vi "5ChTrigs_ABUT.vi"(4 "xmit ring":i32 min=0 max=4 step=1, 5 "Trans Geometry (mm)":T1={"Transducer"=0, "Geo Focus"=12.0, "a (radius)"=3.0, "# of rings"=5, "kerf space "=0.1, "Center Freq"=12.0} {"Transducer" items=["6D 12R 40 MHz"=0, "10D 31R 20 MHz"=1, "10D 23R 20 MHz"=2, "6D 23R 40 MHz"=3, "4.5D 10.7R 40 MHz"=4, "9D 23.5R 20 MHz"=5, "9D 25.8R 20MHz"=6, "Enter"=99]}, 6 "Digitizer Settings":T3={"Digitizer delay (us) "=0.0, "rf points per line"=2048, "lines per plane"=128, "Samp Rate (Hz)"=100000000.0, "Additional dig delay (us)"=0.0, "Voltage Scale"=0.4, "Pre-Looks"=0, "Offset delay (us)"=0.0, "bits A/D"=8, "Avg Num"=1, "DigTimeOut"=5.0, "Rel Dig Delay"=0.0, "Dig Ch"=0, "LeCroyCluster"={"LeCroy Channels"=[TRUE, FALSE, FALSE, FALSE], "LC read pt offset"=0.0, "Sweep Avg"=FALSE}, "Main Digitizer"=enum."NI Digitizer", "Dig Config"=enum."Single channel", "Digitizer ID Cluster"={"Acqiris/Alazar/SP ID"=[], "NI Instr Handles"=[], "LeCroy VISA"="", "GaGe Handle"={"Handle"=0, "Sample size"=0, "Resolution"=0, "Offset"=0, "Channels"=0, "Boards"=0}, "ATS Ref"="ATS9350", "Acqiris Address"=["PCI::INSTR0"], "ADQRef"=refnum, "adq_cu_ptr"=refnum}, "Trigger Settings"={"Trig Source"=1, "Trig Coupling"=0, "Trig Slope"=0, "Level (mV)"=1500.0}, "Bulk Acq"=FALSE, "Bulk Start Indexes"=[], "Data Ref RF"=refnum, "NI ID/Channel"=[], "Total Dig CH"=1, "Xtra Ann Trig delay (us)"=10.0, "Fix Z Delay?"=FALSE, "One Way Transmission?"=FALSE, "Data Ref Log"=refnum} {"Trigger Settings"."Trig Slope" items=["Positive", "Negative"]; "Trigger Settings"."Level (mV)" format="%.2f"; "Trigger Settings"."Trig Coupling" items=["DC 1 MOhm", "AC 1 MOhm", "DC 50 Ohm", "AC 50 Ohm"]; "Trigger Settings"."Trig Source" items=["Chan 1", "External"]; "Rel Dig Delay" format="%.2f"; "DigTimeOut" format="%.2f"; "Avg Num" min=1; "Offset delay (us)" format="%.2f"; "Additional dig delay (us)" format="%.2f"; "Digitizer delay (us)" format="%.2f"}, 7 "high time":dbl=5e-06 format="%^.2e", 8 "Alt trig?":bool, 9 "M-mode?":bool, 10 "error in":errorcluster) -> (0 "5CH Pulser Tasks":refnum<k21>[](array[refnum]), 3 "error out":errorcluster)   [LabVIEW 2022 SP3]
uses:
  Digitizers/-DigitizerRoutines/DigitizerSettings.ctl
  Digitizers/-DigitizerRoutines/Digitizer.ctl
  Digitizers/-DigitizerRoutines/DigConfig.ctl
  Digitizers/-DigitizerRoutines/DigitizerID.ctl
  C:/Windows/System32/ADQAPI_dotNet_helper.dll
  Annular Array/-AnnularRoutines/TransGeometry.ctl
  Annular Array/-AnnularRoutines/ArrayGeometry.ctl
  Motion Controllers/-MotionRoutines/MotionGlobals.vi
  <vilib>/DAQmx/create/channels.llb/DAQmx Create Channel (CO-Pulse Generation-Time).vi
  <vilib>/DAQmx/configure/trigger.llb/DAQmx Start Trigger (Digital Edge).vi
  PulserGlobals.vi
  <vilib>/DAQmx/create/channels.llb/DAQmx Create Channel (CO-Pulse Generation-Frequency).vi
  <vilib>/DAQmx/configure/timing.llb/DAQmx Timing (Implicit).vi
  <resource>/objmgr/daqmx.rc
panel:
  out "time delay (s)":sgl[][](array[numeric])
  out "FZones (m)":dbl[](array[numeric])
  in  "stop":bool
  # "Trigger source comes from Gate of CTR0 (PFI9)\n\nThe NI trigger connector routes to CTR0 Gate"
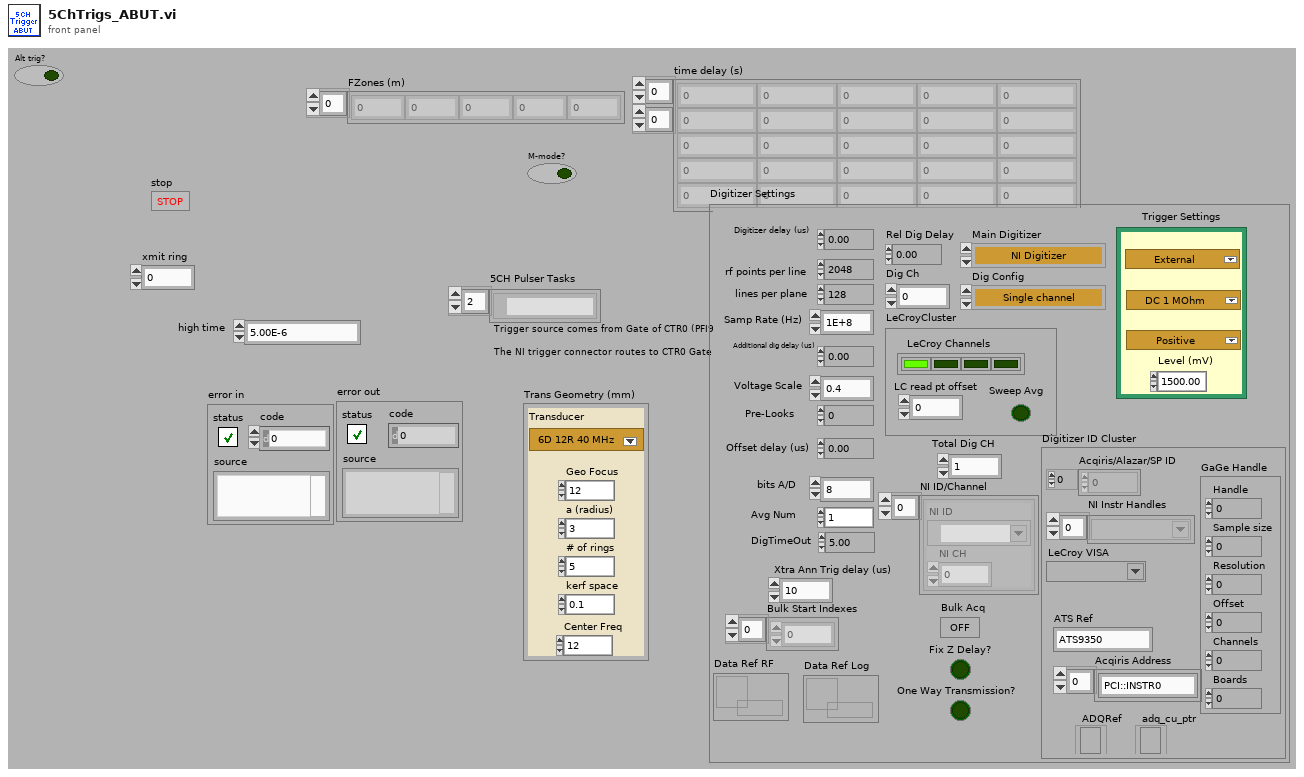
[diagram p1: front panel]
types:
  T1 = typedef "TransGeometry.ctl" = cluster{"Transducer":T2, "Geo Focus":dbl, "a (radius)":dbl, "# of rings":i32, "kerf space ":dbl, "Center Freq":dbl}
  T2 = typedef "ArrayGeometry.ctl" = u16
  T3 = typedef "DigitizerSettings.ctl" = cluster{"Digitizer delay (us) ":dbl, "rf points per line":i32, "lines per plane":i32, "Samp Rate (Hz)":dbl, "Additional dig delay (us)":dbl, "Voltage Scale":dbl, "Pre-Looks":i32, "Offset delay (us)":dbl, "bits A/D":i8, "Avg Num":i32, "DigTimeOut":sgl, "Rel Dig Delay":sgl, "Dig Ch":i32, "LeCroyCluster":cluster{"LeCroy Channels":bool[], "LC read pt offset":dbl, "Sweep Avg":bool}, "Main Digitizer":T4, "Dig Config":T5, "Digitizer ID Cluster":T6, "Trigger Settings":cluster{"Trig Source":u16, "Trig Coupling":u16, "Trig Slope":u16, "Level (mV)":dbl}, "Bulk Acq":bool, "Bulk Start Indexes":i32[], "Data Ref RF":refnum<data-value>, "NI ID/Channel":cluster{"NI ID":refnum<k15>, "NI CH":i32}[], "Total Dig CH":i32, "Xtra Ann Trig delay (us)":dbl, "Fix Z Delay?":bool, "One Way Transmission?":bool, "Data Ref Log":refnum<data-value>}
  T4 = typedef "Digitizer.ctl" = enum16{"Acqiris Digitizer", "NI Digitizer", "LeCroy", "GaGe", "AlazarTech", "No Digitizer", "Teledyne"}
  T5 = typedef "DigConfig.ctl" = enum16{"Single channel", "2 Chans w/ 2 Acqiris", "2 Chans w/ 1 Acqiris", "5-CH Pulser New", "5-CH pulser w/ ann array", "5-pass style ann array", "Empty"}
  T6 = typedef "DigitizerID.ctl" = cluster{"Acqiris/Alazar/SP ID":u32[], "NI Instr Handles":refnum<k15>[], "LeCroy VISA":refnum<visa-resource-name>, "GaGe Handle":cluster{"Handle":u32, "Sample size":u32, "Resolution":i32, "Offset":i32, "Channels":u32, "Boards":u32}, "ATS Ref":string, "Acqiris Address":string[], "ADQRef":refnum<k24>, "adq_cu_ptr":refnum<k24>}
  T7 = typedef "location.ctl" = enum16{"Automatic", "WCM Main", "Hawaii", "Columbia MM3000", "Columbia  NI System", "NYU", "RRI 2", "UHI Allen", "CUMC RT", "Chiba", "Stony Brook", "WCM Microscopy", "WCM Aeoretch", "WCM Optics Lab", "WCM Main 2Axis", "WCM Rotation", "WCM SAM SMAC", "SERI GP"}
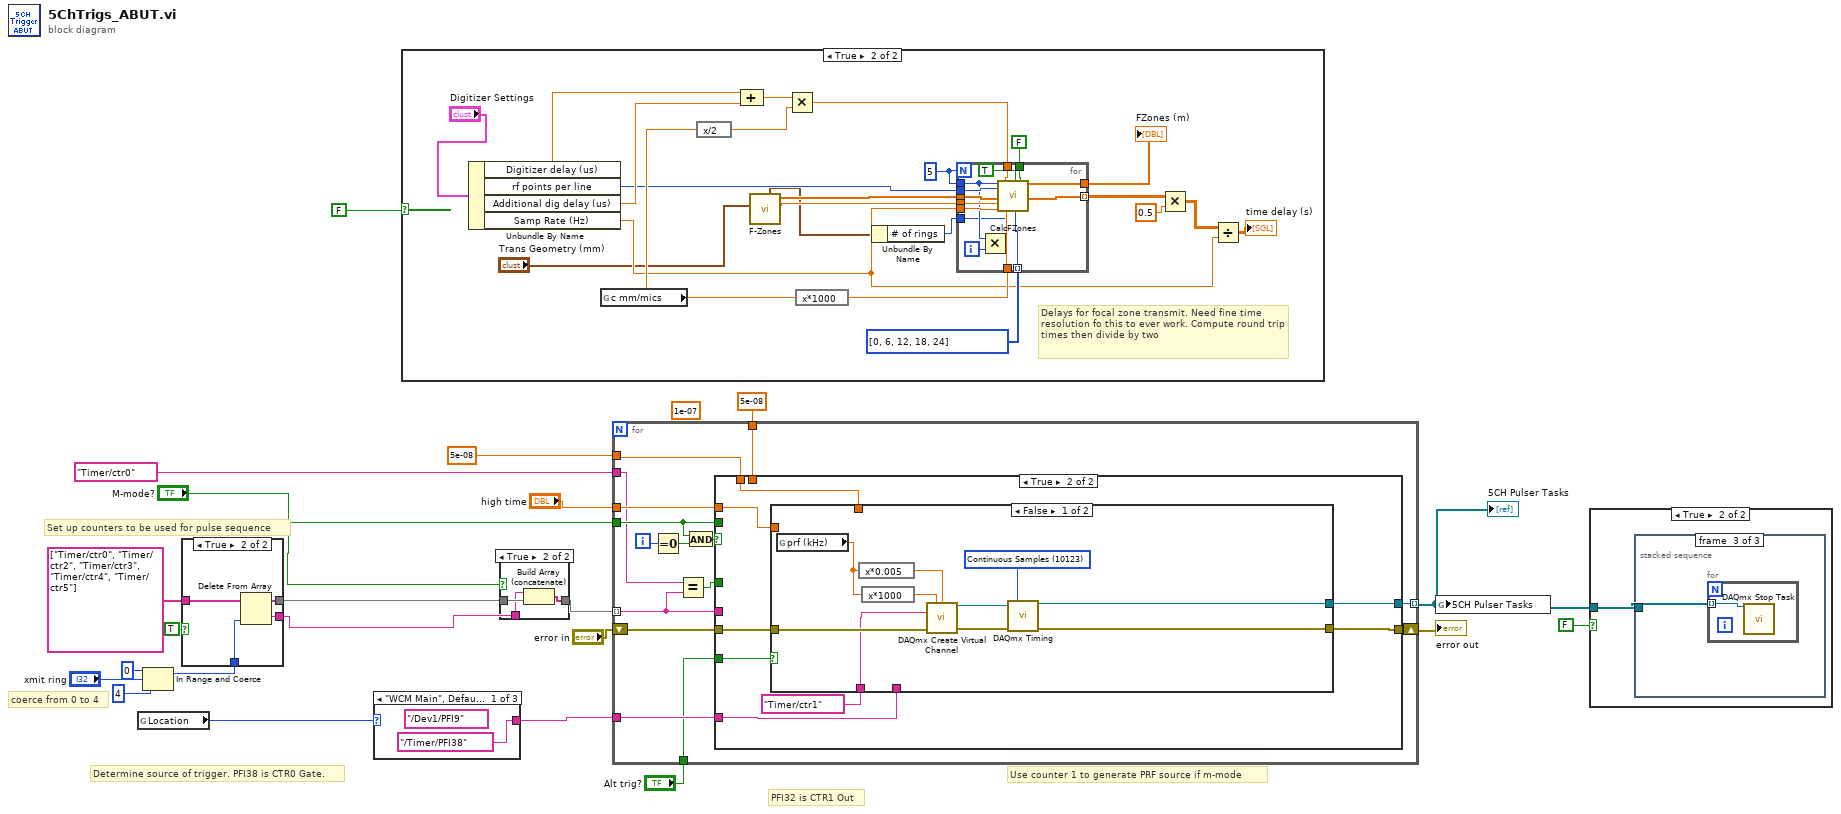
[diagram p0: block diagram]
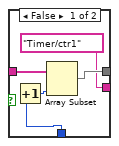
[diagram p2: hidden frame]
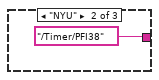
[diagram p5: hidden frame]
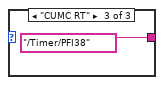
[diagram p6: hidden frame]
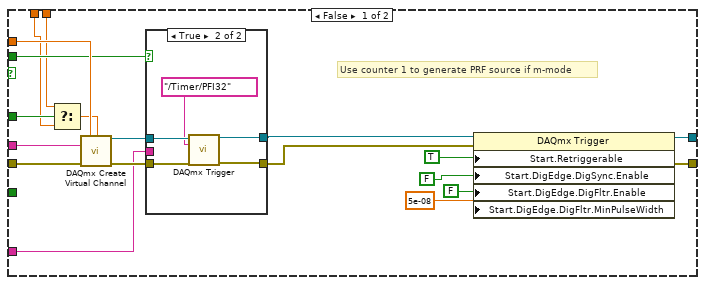
[diagram p7: hidden frame]
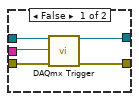
[diagram p8: hidden frame]
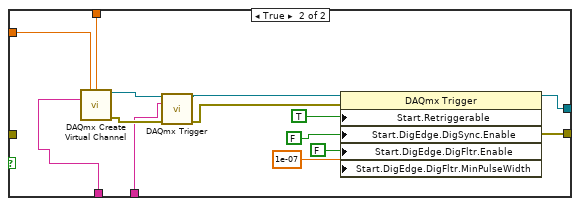
[diagram p9: hidden frame]
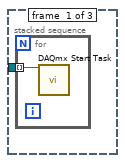
[diagram p11: hidden frame]
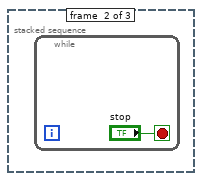
[diagram p12: hidden frame]
diagram:
  (unwired) 1e-07 ("x")
  # "PFI32 is CTR1 Out"
  # "Use counter 1 to generate PRF source if m-mode"
  # "Determine source of trigger. PFI38 is CTR0 Gate."
  # "coerce from 0 to 4"
  # "Set up counters to be used for pulse sequence"
  n1 = global read "MotionGlobals.vi" "Location"() -> (w14:T7)
  n2 = In Range and Coerce(upper limit=0, x="xmit ring", lower limit=4) -> (coerced(x)=w13:i32)  [unwired: 1 out]
  n3 = case shown="True" TRUE {
    tunnel: w13 -> [w23 w31]
    tunnel: [tag "Timer/ctr1" ("Counter(s)") w30] -> w9
    tunnel: tag[] ["Timer/ctr0", "Timer/ctr2", "Timer/ctr3", "Timer/ctr4", "Timer/ctr5"] -> [w27 w29]
    tunnel: [w26 w28] -> w4
    frame False {
      n4 = Increment(x=w23) -> (x+1=w24:i32)
      n5 = Array Subset(array=w27, length=w24) -> (w26:tag[])  [unwired: 1 in]
    }
    frame True {
      n6 = Delete From Array(array=w29, index=w31) -> (deleted portion=w30:tag, array with subset deleted=w28:tag[])  [unwired: 1 in]
    }
  }
  n7 = case shown="\"WCM Main\", Default" w14 {
    tunnel: [tag "/Timer/PFI38" ("Source") tag "/Timer/PFI38" ("Source") tag "/Timer/PFI38" ("Source")] -> w12
    frame "WCM Main", Default {
      (unwired) tag "/Dev1/PFI9" ("Source")
    }
    frame "NYU" {
    }
    frame "CUMC RT" {
    }
  }
  n8 = case shown="True" FALSE {
    frame False {
    }
    frame True {
      w50 = i16 5 ("F- zones")
      # "Delays for focal zone transmit. Need fine time resolution fo this to ever work. Compute round trip times then divide by two"
      n9 = Unbundle By Name("Digitizer Settings") -> ("Digitizer delay (us)"=w42:dbl, "rf points per line"=w39:i32, "Additional dig delay (us)"=w41:dbl, "Samp Rate (Hz)"=w40:dbl)
      n10 = global read "MotionGlobals.vi" "c mm/mics"() -> (w55:sgl)
      n11 = expression code="x/2"(w55) -> (w53:sgl)
      n12 = Compound Arithmetic op=ADD(w42, w41) -> (w54:dbl)
      n13 = call "F-Zones.vi"("Trans Geometry (mm)"="Trans Geometry (mm)") -> ("ROC (m)"=w43:dbl, "annuli rad (m)"=w44:dbl[], "Trans Geometry (mm) out"=w37:T1)  [unwired: 7 in, 1 out]
      n14 = Multiply(x=w54, y=w53) -> (x*y=w52:dbl)
      n15 = expression code="x*1000"(w55) -> (w56:sgl)
      n16 = Unbundle By Name(w37) -> ("# of rings"=w36:i32)
      n17 = for {
        N: w50 -> [_]
        tunnel: w50 -> [w61]
        tunnel: w44 -> [w71]
        tunnel: w43 -> [w70]
        tunnel: w40 -> [w69]
        tunnel: FALSE ("One Way Receive") -> [w68]
        tunnel: w39 -> [w67]
        tunnel: w56 -> [w66]
        tunnel: w52 -> [w65]
        tunnel: [w64] -> w48 mode=indexing
        tunnel: [w63] -> w51
        tunnel: i32[] [0, 6, 12, 18, 24] -> [w59] mode=indexing
        tunnel: w36 -> [w58]
        i -> [w60]
        n18 = Multiply(x=w61, y=w60) -> ()  [unwired: 1 out]
        n19 = call "CalcFZones.vi"("F- zones"=w61, "# rf points per line"=w67, "Radii (m)"=w71, "ROC (m)"=w70, "Sampling Rate"=w69, "delay (mm)"=w65, "# Elements"=w58, "c (m/s)"=w66, "Round to ROC?"=TRUE, "File index number"=w59, "One Way Receive"=w68) -> ("FZones (m)"=w63:dbl[], "ZoneShift"=w64:sgl[])  [unwired: 3 in, 4 out]
      }
      "FZones (m)" <- w51
      n20 = Multiply(x=w48, y=0.5) -> (x*y=w46:dbl[][])
      n21 = Divide(x=w46, y=w40) -> (x/y=→"time delay (s)":dbl[][])
    }
  }
  n22 = case shown="True" "M-mode?" {
    tunnel: [w72 w74] -> w11
    tunnel: w4 -> [w72 w75]
    tunnel: w9 -> [_ w73]
    frame False {
    }
    frame True {
      n23 = Build Array (concatenate)(w73, w75) -> (w74:tag[])
    }
  }
  n24 = for {
    tunnel: "high time" -> [w88]
    shift-right: [w89] -> w22
    shift-left: "error in" -> [w90]
    tunnel: 5e-08 ("x") -> [w81]
    tunnel: w12 -> [w87]
    tunnel: w11 -> [w80] mode=indexing
    tunnel: [w86] -> w15 mode=indexing
    tunnel: "M-mode?" -> [w83]
    tunnel: tag "Timer/ctr0" ("Counter(s)") -> [w79]
    tunnel: 5e-08 ("x") -> [w77]
    tunnel: "Alt trig?" -> [w76]
    i -> [w84]
    n25 = Equal To 0?(x=w84) -> (x = 0?=w82:bool)
    n26 = Equal?(x=w79, y=w80) -> (x = y?=w78:bool)
    n27 = And(x=w83, y=w82) -> (x .and. y?=w85:bool)
    n28 = case shown="True" w85 {
      tunnel: w90 -> [w109 w127]
      tunnel: [w107 w125] -> w89
      tunnel: w80 -> [w106 _]
      tunnel: w88 -> [w104 w122]
      tunnel: w87 -> [w103 w123]
      tunnel: [w102 w126] -> w86
      tunnel: w83 -> [w101 _]
      tunnel: w81 -> [w95 w121]
      tunnel: w78 -> [w98 _]
      tunnel: w77 -> [w96 _]
      tunnel: w76 -> [_ w120]
      frame False {
        # "Use counter 1 to generate PRF source if m-mode"
        n29 = Select(t=w96, s=w98, f=w95) -> (s? t:f=w97:dbl)
        n30 = call-poly <vilib>:"DAQmx Create Virtual Channel.vi"("high time"=w104, "low time"=w97, "counter"=w106, "error in"=w109) -> ("task out"=w105:refnum<k21>, "error out"=w108:errorcluster)  [unwired: 5 in, 5 out]
        n31 = case shown="True" w101 {
          tunnel: w108 -> [w113 w119]
          tunnel: w105 -> [w114 w118]
          tunnel: [w112 w117] -> w100
          tunnel: w103 -> [w110 _]
          tunnel: [w111 w115] -> w99
          frame False {
            n32 = call-poly <vilib>:"DAQmx Trigger.vi"("task/channels in"=w114, "source"=w110, "error in"=w113) -> ("task out"=w112:refnum<k21>, "error out"=w111:errorcluster)  [unwired: 2 in, 9 out]
          }
          frame True {
            n33 = call-poly <vilib>:"DAQmx Trigger.vi"("task/channels in"=w118, "source"=tag "/Timer/PFI32", "error in"=w119) -> ("task out"=w117:refnum<k21>, "error out"=w115:errorcluster)  [unwired: 1 in, 10 out]
          }
        }
        n34 = property class="DAQmx Trigger"(reference=w100, error in=w99, "Start.Retriggerable"=TRUE, "Start.DigEdge.DigSync.Enable"=FALSE, "Start.DigEdge.DigFltr.Enable"=FALSE, "Start.DigEdge.DigFltr.MinPulseWidth"=5e-08) -> (reference out=w102:refnum<k21>, error out=w107:errorcluster)
      }
      frame True {
        n35 = case shown="False" w120 {
          tunnel: w127 -> [w134 _]
          tunnel: [w131 w138] -> w126
          tunnel: [w130 w139] -> w125
          tunnel: tag "Timer/ctr1" ("Counter(s)") -> [w129 w147]
          tunnel: w123 -> [_ w144]
          tunnel: w122 -> [_ w141]
          tunnel: w121 -> [_ w140]
          frame False {
            w137 = 10123 items=["Finite Samples"=10178, "Continuous Samples"=10123, "Hardware Timed Single Point"=12522] ("sample mode")
            n36 = global read "PulserGlobals.vi" "prf (kHz)"() -> (w128:dbl)
            n37 = expression code="x*0.005"(w128) -> (w133:dbl)
            n38 = expression code="x*1000"(w128) -> (w132:dbl)
            n39 = call-poly <vilib>:"DAQmx Create Virtual Channel.vi"("frequency"=w132, "duty cycle"=w133, "counter"=w129, "error in"=w134) -> ("task out"=w136:refnum<k21>, "error out"=w135:errorcluster)  [unwired: 6 in, 4 out]
            n40 = call-poly <vilib>:"DAQmx Timing.vi"("task/channels in"=w136, "sample mode"=w137, "error in"=w135) -> ("task out"=w131:refnum<k21>, "error out"=w130:errorcluster)  [unwired: 11 in]
          }
          frame True {
            n41 = call-poly <vilib>:"DAQmx Create Virtual Channel.vi"("high time"=w141, "low time"=w140, "counter"=w147) -> ("task out"=w146:refnum<k21>, "error out"=w145:errorcluster)  [unwired: 6 in, 5 out]
            n42 = call-poly <vilib>:"DAQmx Trigger.vi"("task/channels in"=w146, "source"=w144, "error in"=w145) -> ("task out"=w143:refnum<k21>, "error out"=w142:errorcluster)  [unwired: 2 in, 9 out]
            n43 = property class="DAQmx Trigger"(reference=w143, error in=w142, "Start.Retriggerable"=TRUE, "Start.DigEdge.DigSync.Enable"=FALSE, "Start.DigEdge.DigFltr.Enable"=FALSE, "Start.DigEdge.DigFltr.MinPulseWidth"=1e-07) -> (reference out=w138:refnum<k21>, error out=w139:errorcluster)
          }
        }
      }
    }
  }
  "error out" <- w22
  "5CH Pulser Tasks" <- w15
  n44 = global write "MotionGlobals.vi" "5CH Pulser Tasks"(w15) -> ()
  n45 = case shown="True" FALSE {
    tunnel: w15 -> [_ w152]
    frame False {
    }
    frame True {
      n46 = stacked-sequence {
        tunnel: w152 -> [w153 _ w156]
        frame #0 {
          n47 = for {
            tunnel: w153 -> [w154] mode=indexing
            n48 = call <vilib>:"DAQmx Start Task.vi"("task/channels in"=w154) -> ()  [unwired: 13 in, 2 out]
          }
        }
        frame #1 {
          n49 = while {
            stop <- "stop" stop-if-true
          }
        }
        frame #2 {
          n50 = for {
            tunnel: w156 -> [w157] mode=indexing
            n51 = call <vilib>:"DAQmx Stop Task.vi"("task/channels in"=w157) -> ()  [unwired: 13 in, 2 out]
          }
        }
      }
    }
  }
